vi "WiiBalanceBoard_Write_LED.vi"(2 "error in":errorcluster, 3 "Balance Board LED":bool, 4 "hWiimoteHandle in":u32) -> (0 "error out":errorcluster, 1 "hWiimoteHandle out":u32)   [LabVIEW 2010]
doc: "CETPD\nActivate/desactivate the button LED"
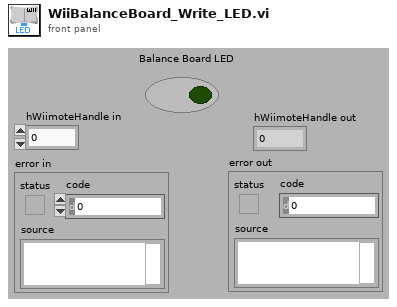
[diagram p1: front panel]
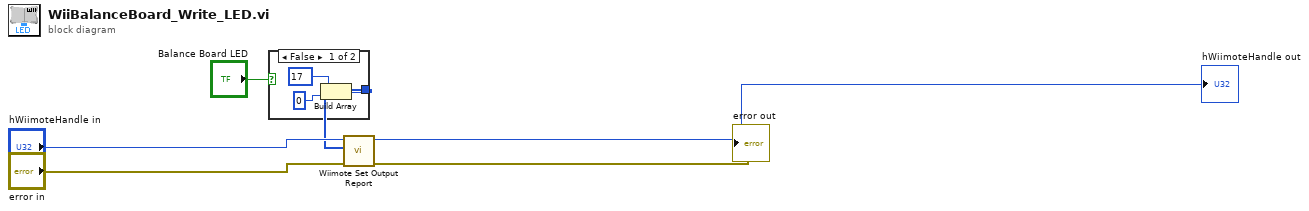
[diagram p0: block diagram]
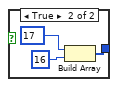
[diagram p2: hidden frame]
diagram:
  n1 = case shown="False" "Balance Board LED" {
    tunnel: [w7 w10] -> w2
    frame False {
      n2 = Build Array(u8 17, u8 0 ("element")) -> (w7:u8[])
    }
    frame True {
      n3 = Build Array(u8 17, u8 16 ("element")) -> (w10:u8[])
    }
  }
  n4 = call "Wiimote Set Output Report.vi"("error in"="error in", "pReportBuffer in"=w2, "hWiimoteHandle in"="hWiimoteHandle in") -> ("error out"=→"error out":errorcluster, "hWiimoteHandle out"=→"hWiimoteHandle out":u32)  [unwired: 7 in]
